vi "_check_attribute_for_writing.vi"(6 "Expected Data Type":T1, 7 "Attribute":T2={"Identifier"="", "Descriptive Name"="", "Data Type"=enum."Integer 32", "Command"="", "Access"=enum."Read/Write", "Range Table"="", "Read Callback"="", "Write Callback"="", "Supported Models"="", "Instrument Options"="", "Index"=0, "OPC Wait"=FALSE, "No Status Check"=FALSE, "Cache Only"=FALSE}, 8 "error in":errorcluster caption="error in (no error)", 11 "VISA resource name":refnum<visa-resource-name>) -> (0 "error out":errorcluster, 3 "VISA resource name out":refnum<visa-resource-name>)   [LabVIEW 2022 SP3, in "hmp4000_rsidr_core.lvlib"]
uses:
  hmp4000_rsidr_core.lvlib
  type_Attribute.ctl
  type_Attribute_Data_Type.ctl
  type_ReadWriteAccess.ctl
  type_Error_Codes.ctl
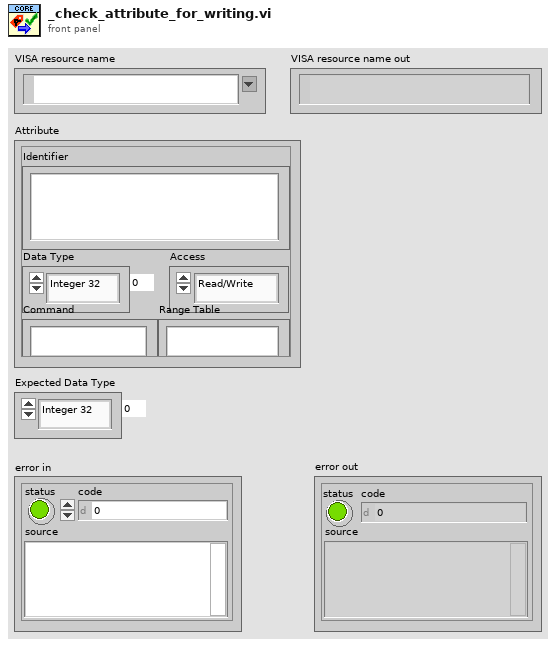
[diagram p1: front panel]
types:
  T1 = typedef "hmp4000_rsidr_core.lvlib/type_Attribute_Data_Type.ctl" = enum16{"Integer 32", "Double", "String", "Boolean", "None", "Integer 64", "RawString"}
  T2 = typedef "hmp4000_rsidr_core.lvlib/type_Attribute.ctl" = cluster{"Identifier":string, "Descriptive Name":string, "Data Type":T1, "Command":string, "Access":T3, "Range Table":string, "Read Callback":string, "Write Callback":string, "Supported Models":string, "Instrument Options":string, "Index":i32, "OPC Wait":bool, "No Status Check":bool, "Cache Only":bool}
  T3 = typedef "hmp4000_rsidr_core.lvlib/type_ReadWriteAccess.ctl" = enum16{"Read Only", "Write Only", "Read/Write"}
  T4 = typedef "hmp4000_rsidr_core.lvlib/type_Error_Codes.ctl" = enum16{"No_error", "VISA_err_ResourceNotFound", "VISA_err_Timeout", "VISA_warn_MoreDataAvailable", "RS_err_MissingCallback", "RS_err_InvalidAttribute", "RS_err_InvalidValue", "RS_err_UnknownResource", "RS_err_AlreadyInitialized", "RS_err_InstrumentStatus", "RS_err_BadRepCapName", "RS_err_TypesMismatch", "RS_err_ValueNotSupported", "RS_err_InvalidRngTable", "RS_err_IDqueryFail", "RS_err_UnexpResponse", "VISA_warn_ConfigNotLoaded", "RS_err_AttributeNotReadable", "RS_err_AttributeNotWritable", "RS_err_InstrumentType", "RS_err_InstrumentOption", "VISA_err_InvalidSize", "RS_err_ReliabilityIndicator", "VISA_warn_UnknownStatus", "VISA_warn_TermCharRead", "VISA_err_IO_error", "RS_err_FunctionNotSupported", "VISA_warn_QueueEmpty"}
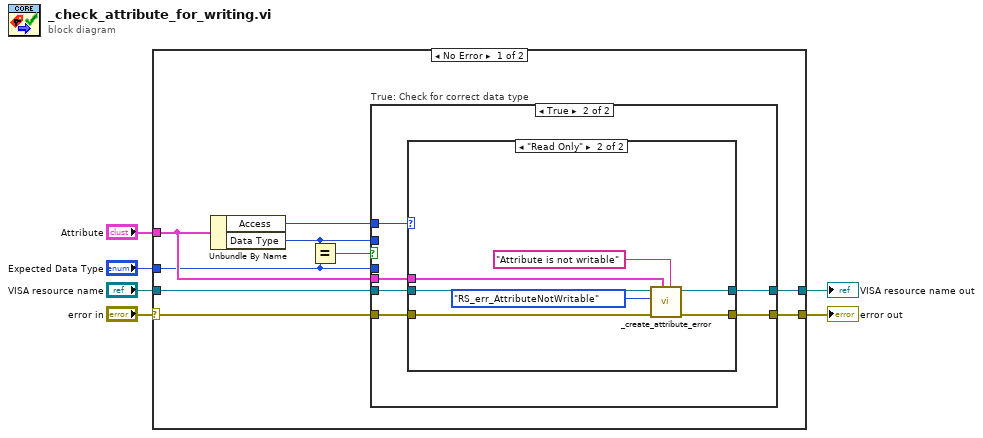
[diagram p0: block diagram]
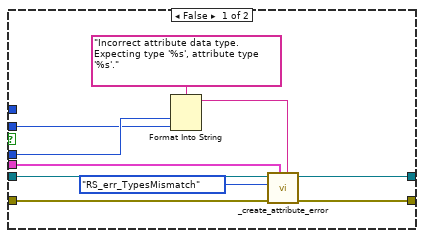
[diagram p2: hidden frame]
diagram:
  n1 = case shown="No Error" "error in" {
    selector: "error in" -> [w12 w42]
    tunnel: [w14 w42] -> w5
    tunnel: "VISA resource name" -> [w10 w41]
    tunnel: [w9 w41] -> w3
    tunnel: "Attribute" -> [w8 _]
    tunnel: "Expected Data Type" -> [w7 _]
    frame No Error {
      n2 = Unbundle By Name(w8) -> ("Access"=w13:T3, "Data Type"=w11:T1)
      n3 = Equal?(x=w11, y=w7) -> (x = y?=w15:bool)
      n4 = case "True: Check for correct data type" shown="True" w15 {
        tunnel: [w25 w28] -> w14
        tunnel: w13 -> [_ w31]
        tunnel: w12 -> [w24 w30]
        tunnel: w8 -> [w21 w26]
        tunnel: w7 -> [w17 _]
        tunnel: w11 -> [w16 _]
        tunnel: w10 -> [w20 w29]
        tunnel: [w18 w27] -> w9
        frame False {
          n5 = Format Into String(format string="Incorrect attribute data type. Expecting type '%s', attribute type '%s'.", w17, w16) -> (resulting string=w22:string)  [unwired: 2 in, 1 out]
          n6 = call "_create_attribute_error.vi"("Error Elaboration (\"\")"=w22, "Attribute"=w21, "error in"=w24, "Error Enum in"=type_Error_Codes."RS_err_TypesMismatch" ("Error Enum in (from err to recompose)"), "VISA resource name"=w20) -> ("error out"=w25:errorcluster, "VISA resource name out"=w18:refnum<visa-resource-name>)  [unwired: 5 in]
        }
        frame True {
          n7 = case shown="\"Read Only\"" w31 {
            tunnel: w30 -> [w33 w39]
            tunnel: w29 -> [w32 w38]
            tunnel: [w33 w37] -> w28
            tunnel: [w32 w36] -> w27
            tunnel: w26 -> [_ w34]
            frame "Write Only", "Read/Write" {
            }
            frame "Read Only" {
              n8 = call "_create_attribute_error.vi"("Error Elaboration (\"\")"="Attribute is not writable" ("string"), "Attribute"=w34, "error in"=w39, "Error Enum in"=type_Error_Codes."RS_err_AttributeNotWritable" ("Error Enum in (from err to recompose)"), "VISA resource name"=w38) -> ("error out"=w37:errorcluster, "VISA resource name out"=w36:refnum<visa-resource-name>)  [unwired: 5 in]
            }
          }
        }
      }
    }
    frame Error {
    }
  }
  "VISA resource name out" <- w3
  "error out" <- w5
